vi "Get Reply Protocol.vi"(8 "Error In":errorcluster, 10 "Identifier":string, 11 "reference in":refnum<class "Reply Protocol Manager.lvclass">) -> (0 "Error Out":errorcluster, 2 "Reply Protocol Base":refnum<class "Reply Protocol Base.lvclass">, 3 "reference out":refnum<class "Reply Protocol Manager.lvclass">)   [LabVIEW 2023, in "HAL GOOP4.lvlib" / "Reply Protocol Manager.lvclass"]
uses:
  Reply Protocol Manager.lvclass
  Reply Protocol Manager.lvclass/Reply Protocol Manager.ctl
  Reply Protocol/Reply Protocol Base/Reply Protocol Base.lvclass
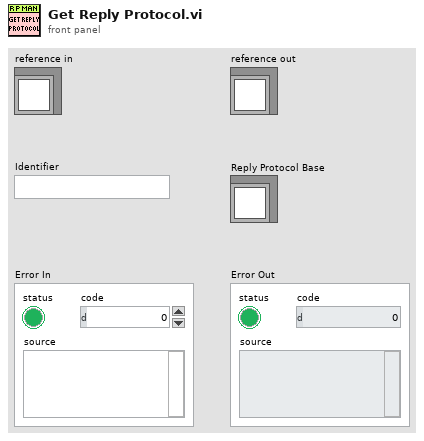
[diagram p1: front panel]
types:
  T1 = typedef "HAL GOOP4.lvlib/Reply Protocol Manager.lvclass/ObjectAttributes.ctl" = cluster{"Reply Protocols":map{string, refnum<class "Reply Protocol Base.lvclass">}}
  T2 = map{string, refnum<class "Reply Protocol Base.lvclass">}
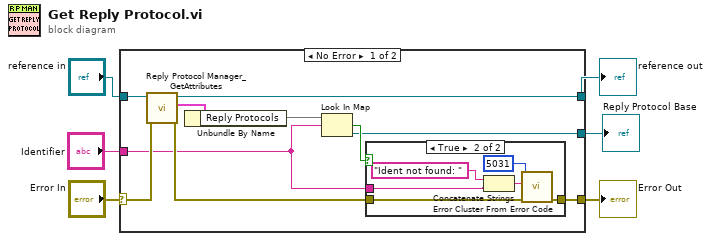
[diagram p0: block diagram]
diagram:
  n1 = case shown="No Error" "Error In" {
    selector: "Error In" -> [w16 w25]
    tunnel: [w11 w25] -> w5
    tunnel: [w13 w24] -> w3
    tunnel: "reference in" -> [w14 w24]
    tunnel: "Identifier" -> [w7 _]
    tunnel: [w8 _] -> w1
    frame No Error {
      n2 = call "Reply Protocol Manager_GetAttributes.vi"("Error In"=w16, "reference in"=w14) -> ("Error Out"=w9:errorcluster, "Data"=w15:T1, "reference out"=w13:refnum<class "Reply Protocol Manager.lvclass">)  [unwired: 6 in, 1 out]
      n3 = Unbundle By Name(w15) -> ("Reply Protocols"=w12:T2)
      n4 = Look In Map(map=w12, key=w7) -> (key not found?=w10:bool, value=w8:refnum<class "Reply Protocol Base.lvclass">)  [unwired: 1 in]
      n5 = case shown="True" w10 {
        tunnel: [w17 w23] -> w11
        tunnel: w9 -> [w17 w22]
        tunnel: w7 -> [_ w19]
        frame False {
        }
        frame True {
          n6 = Concatenate Strings("Ident not found: " ("error message (\"\")"), w19) -> (w20:string)
          n7 = call <vilib>:"Error Cluster From Error Code.vi"("error in (no error)"=w22, "error message (\"\")"=w20, "error code (0)"=5031) -> ("error out"=w23:errorcluster)  [unwired: 6 in]
        }
      }
    }
    frame Error {
    }
  }
  "Error Out" <- w5
  "reference out" <- w3
  "Reply Protocol Base" <- w1
